vi "Teleop.vi"(10 "Match Info":T1={"Autonomous Elapsed Seconds"=0.0, "TeleOp Elapsed Seconds"=31.144, "Disabled Elapsed Seconds"=2.36, "Visited Autonomous"=FALSE, "Visited TeleOp"=TRUE, "Visited Disabled"=TRUE, "Autonomous Settings"={"Autonomous Style"=enum."Independent", "VI Refnum"=refnum}}, 11 "Call Context":T2=enum."Stop") -> ()   [LabVIEW 2018]
doc: "This VI is called for each TeleOp packet received from the DS where the robot is not disabled. It is often used to read from the joysticks and update I/O or to update setpoints for timed control loops. It should complete and return within 20 milliseconds or it may miss DS packets."
uses:
  <vilib>/Rock Robotics/WPI/DriverStation/WPI_DriverStationDerivedRobotMode.ctl
  <vilib>/Rock Robotics/WPI/DriverStation/WPI_DriverStationMatch Info.ctl
  <vilib>/Rock Robotics/WPI/Utilities/WPI_GetSetVariantRefNum.vi
  <vilib>/Rock Robotics/Network Tables/NT Read Numeric Array.vi
  <vilib>/Rock Robotics/Network Tables/NT Read Boolean.vi
  Robot Global Data.vi
  <vilib>/Rock Robotics/WPI/ThirdParty/Phoenix-LabVIEW/Motor Controller/Get/CTRE_Phoenix_MotorController_GetSelectedSensorData.vi
panel:
  out "RightDriveVelocity":i32(graph)
  out "LeftDriveVelocity":i32(graph)
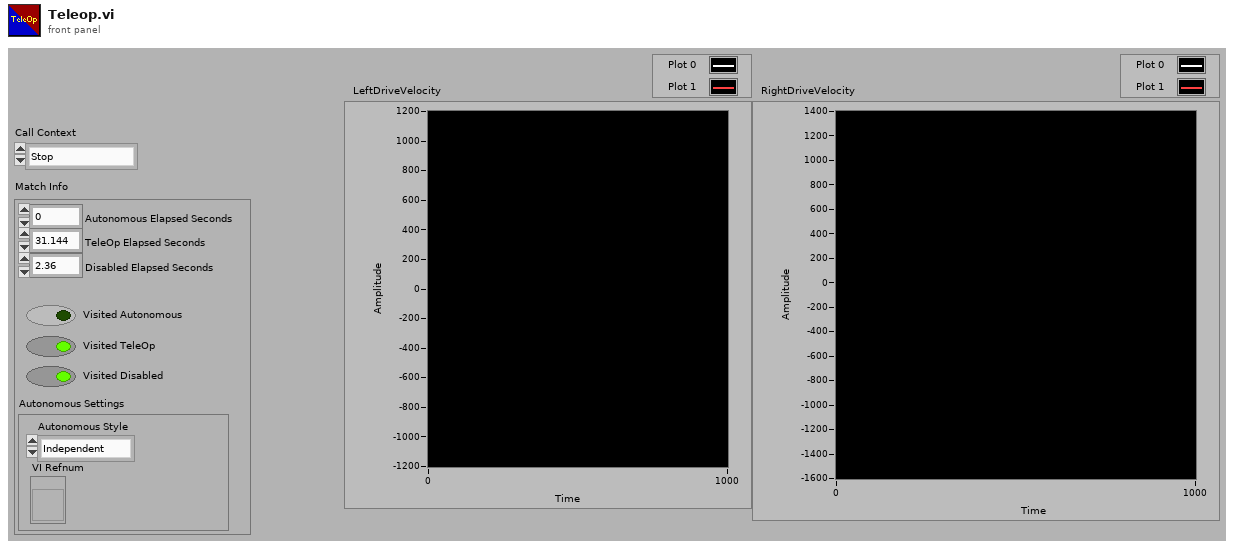
[diagram p1: front panel]
types:
  T1 = typedef "WPI_DriverStationMatch Info.ctl" = cluster{"Autonomous Elapsed Seconds":dbl, "TeleOp Elapsed Seconds":dbl, "Disabled Elapsed Seconds":dbl, "Visited Autonomous":bool, "Visited TeleOp":bool, "Visited Disabled":bool, "Autonomous Settings":cluster{"Autonomous Style":enum16{"Iterative", "Independent"}, "VI Refnum":refnum<vi>}}
  T2 = typedef "WPI_DriverStationDerivedRobotMode.ctl" = enum16{"Init", "Execute", "Stop"}
  T3 = typedef "WPI_JoystickDevRef.ctl" = cluster{"Device":T4}
  T4 = typedef "WPI_JoystickDeviceEnum.ctl" = enum16{"USB 0", "USB 1", "USB 2", "USB 3", "USB 4", "USB 5"}
  T5 = typedef "WPI_MotorControlDeviceRef.ctl" = cluster{"DeviceStatus":errorcluster, "Type":T6, "PWM":cluster{"PWM Channel":T7, "DeadBand":T8}, "CAN":cluster{"Device Number":u8, "SetOutput VI Ref":variant, "GetOutput VI Ref":variant, "Enable VI Ref":variant, "Disable VI Ref":variant, "Data":variant}, "Invert":bool, "DIO PWM":cluster{"PWM \"Enable\" Channel":T7, "DIOChannel":T9, "PWM Rate":dbl}}
  T6 = typedef "WPI_MotorControlType.ctl" = enum16{"PWM", "CAN", "DIO PWM"}
  T7 = typedef "FPGA_DIOPWMChannel.ctl" = enum8{"PWM 0", "PWM 1", "PWM 2", "PWM 3", "PWM 4", "PWM 5", "PWM 6", "PWM 7", "PWM 8", "PWM 9", "PWM MXP 0", "PWM MXP 1", "PWM MXP 2", "PWM MXP 3", "PWM MXP 4", "PWM MXP 5", "PWM MXP 6", "PWM MXP 7", "PWM MXP 8", "PWM MXP 9", "Invalid"}
  T8 = typedef "WPI_PWMDeadband.ctl" = cluster{"Name":string, "maxPositivePwm":i32, "minPositivePwm":i32, "centerPwm":i32, "maxNegativePwm":i32, "minNegativePwm":i32, "angularRange":u16}
  T9 = typedef "FPGA_DIOChannel.ctl" = enum8{"DIO 0", "DIO 1", "DIO 2", "DIO 3", "DIO 4", "DIO 5", "DIO 6", "DIO 7", "DIO 8", "DIO 9", "DIO MXP 0", "DIO MXP 1", "DIO MXP 2", "DIO MXP 3", "DIO MXP 4", "DIO MXP 5", "DIO MXP 6", "DIO MXP 7", "DIO MXP 8", "DIO MXP 9", "DIO MXP 10", "DIO MXP 11", "DIO MXP 12", "DIO MXP 13", "DIO MXP 14", "DIO MXP 15", "SPI Port CS1", "SPI Port CS2", "SPI Port CS3", "SPI Port MISO", "SPI Port MOSI", "Invalid"}
  T10 = typedef "CTRE_Phoenix_MotorControl_ControlMode.ctl" = u16
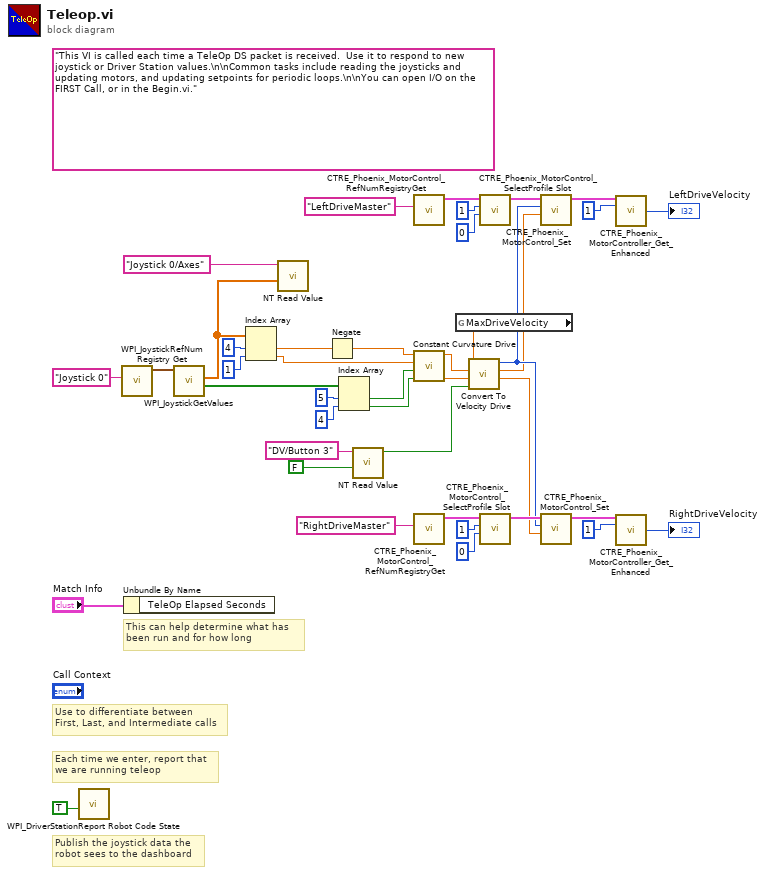
[diagram p0: block diagram]
diagram:
  (unwired) "This VI is called each time a TeleOp DS packet is received.  Use it to respond to new joystick or Driver Station values.\n\nCommon tasks include reading the joysticks and updating motors, and updating setpoints for periodic loops.\n\nYou can open I/O on the FIRST Call, or in the Begin.vi."
  # "Publish the joystick data the\nrobot sees to the dashboard"
  # "Each time we enter, report that\nwe are running teleop"
  # "Use to differentiate between\nFirst, Last, and Intermediate calls"
  # "This can help determine what has\nbeen run and for how long"
  n1 = call <vilib>:"WPI_DriverStationReport Robot Code State.vi"("TeleOp"=TRUE ("Autonomous")) -> ()  [unwired: 10 in, 1 out]
  n2 = call <vilib>:"WPI_JoystickRefNum Registry Get.vi"("refnum name"="Joystick 0") -> ("JoystickDevRef"=w37:T3)  [unwired: 9 in, 1 out]
  n3 = Unbundle By Name("Match Info") -> ()  [unwired: 1 out]
  n4 = call <vilib>:"WPI_JoystickGetValues.vi"("JoystickDevRef"=w37) -> ("Buttons"=w19:bool[], "Axes"=w32:dbl[])  [unwired: 6 in, 3 out]
  n5 = Index Array(array=w32, index #1=4 ("index"), index #2=1 ("index")) -> (element #1=w9:dbl, element #2=w7:dbl)
  n6 = call-poly <vilib>:"NT Read Value.vi"("Default Value"=w32, "Name"="Joystick 0/Axes") -> ()  [unwired: 8 in, 2 out]
  n7 = Negate(x=w9) -> (-x=w8:dbl)
  n8 = Index Array(array=w19, index #1=5 ("index"), index #2=4 ("index")) -> (element #1=w16:bool, element #2=w15:bool)
  n9 = call-poly <vilib>:"NT Read Value.vi"("Default Value"=FALSE, "Name"="DV/Button 3") -> ("Boolean"=w3:bool)  [unwired: 8 in, 1 out]
  n10 = call <vilib>:"CTRE_Phoenix_MotorControl_RefNumRegistryGet.vi"("refnum name"="LeftDriveMaster") -> ("PhoenixMotorControlDevRef"=w27:T5)  [unwired: 9 in, 1 out]
  n11 = call "Constant Curvature Drive.vi"("Turbo?"=w15, "QuickTurn?"=w16, "Speed"=w7, "Curve"=w8) -> ("Right Percent Setpoint"=w13:dbl, "Left Percent Setpoint"=w14:dbl)  [unwired: 6 in]
  n12 = call <vilib>:"CTRE_Phoenix_MotorControl_RefNumRegistryGet.vi"("refnum name"="RightDriveMaster") -> ("PhoenixMotorControlDevRef"=w21:T5)  [unwired: 9 in, 1 out]
  n13 = global read "Robot Global Data.vi" "MaxDriveVelocity"() -> (w1:dbl)
  n14 = call "Convert To Velocity Drive.vi"("Abort Velocity Control"=w3, "Right Percent Output"=w13, "Left Percent Output"=w14, "Max Velocity Physically Allowed"=w1) -> ("Right Output"=w10:dbl, "Left Output"=w11:dbl, "Control Mode"=w12:T10)  [unwired: 5 in]
  n15 = call <vilib>:"CTRE_Phoenix_MotorControl_SelectProfile Slot.vi"("pidLoopIdx"=0, "slotIdx"=1 ("pidLoopIdx"), "PhoenixMotorControlDevRef"=w27) -> ("PhoenixMotorControlDevRef"=w26:T5)  [unwired: 7 in, 1 out]
  n16 = call <vilib>:"CTRE_Phoenix_MotorControl_SelectProfile Slot.vi"("pidLoopIdx"=0, "slotIdx"=1 ("pidLoopIdx"), "PhoenixMotorControlDevRef"=w21) -> ("PhoenixMotorControlDevRef"=w20:T5)  [unwired: 7 in, 1 out]
  n17 = call <vilib>:"CTRE_Phoenix_MotorControl_Set.vi"("Output"=w11, "Control Mode"=w12, "PhoenixMotorControlDevRef"=w26) -> ("PhoenixMotorControlDevRef"=w31:T5)  [unwired: 7 in, 1 out]
  n18 = call <vilib>:"CTRE_Phoenix_MotorControl_Set.vi"("Output"=w10, "Control Mode"=w12, "PhoenixMotorControlDevRef"=w20) -> ("PhoenixMotorControlDevRef"=w29:T5)  [unwired: 7 in, 1 out]
  n19 = call-poly <vilib>:"CTRE_Phoenix_MotorController_Get_Enhanced.vi"("PhoenixMotorControlDevRef"=w31, "pidLoopIdx"=u32 1) -> ("Velocity (Raw Sensor Units per 100 ms)"=→"LeftDriveVelocity":i32)  [unwired: 10 in, 3 out]
  n20 = call-poly <vilib>:"CTRE_Phoenix_MotorController_Get_Enhanced.vi"("PhoenixMotorControlDevRef"=w29, "pidLoopIdx"=u32 1) -> ("Velocity (Raw Sensor Units per 100 ms)"=→"RightDriveVelocity":i32)  [unwired: 10 in, 3 out]
